vi "ExposeFastConvertNetObjToNumericArray.vi"(11 ".NET Refnum in":refnum<k24>) -> (3 "Array":variant)   [LabVIEW 2017]
uses:
  Mapper/ExposeMapperDataTypeEnum.ctl
  C:/Code/CMCryoSysCode/Expose/COM/CSCom/CSCom/bin/Release/CSCom.dll
  COM/CSCom/CSCom/bin/Release/CSCom.dll
  600bb580-dba4-4572-ab6a-3221339fa0df.vi
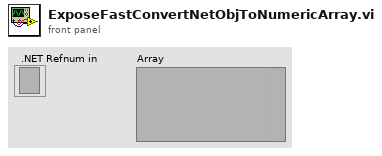
[diagram p1: front panel]
types:
  T1 = typedef "ExposeMapperDataTypeEnum.ctl" = enum16{"NotData", "int8", "byte", "int16", "uint16", "int32", "uint32", "int64", "uint64", "Single", "Double", "String", "Boolean", "Container"}
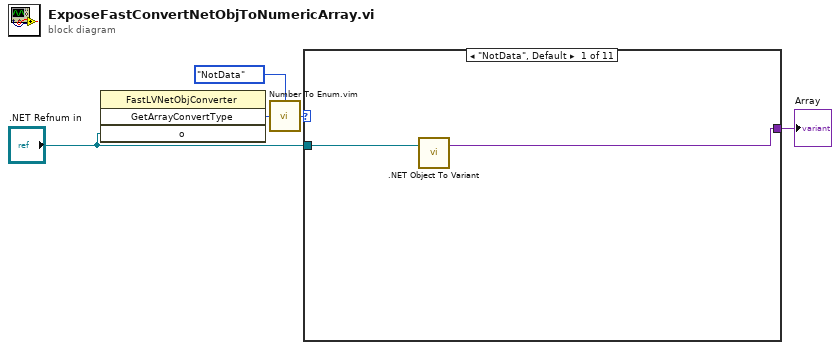
[diagram p0: block diagram]
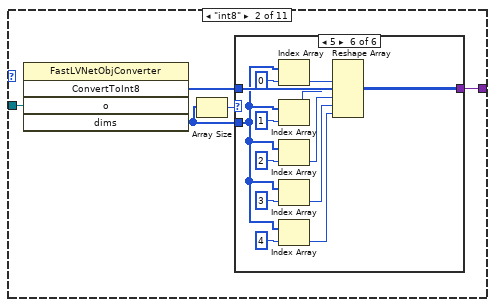
[diagram p2: hidden frame]
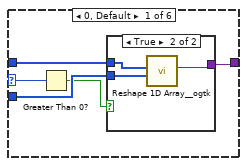
[diagram p3: hidden frame]
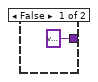
[diagram p4: hidden frame]
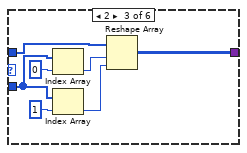
[diagram p6: hidden frame]
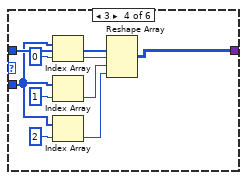
[diagram p7: hidden frame]
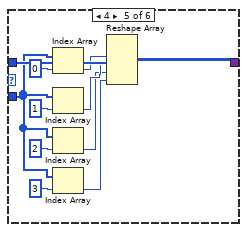
[diagram p8: hidden frame]
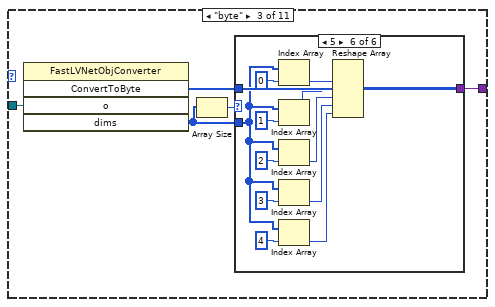
[diagram p9: hidden frame]
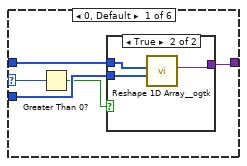
[diagram p10: hidden frame]
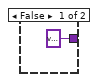
[diagram p11: hidden frame]
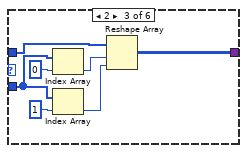
[diagram p13: hidden frame]
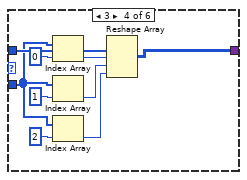
[diagram p14: hidden frame]
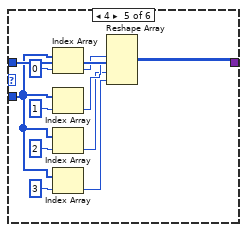
[diagram p15: hidden frame]
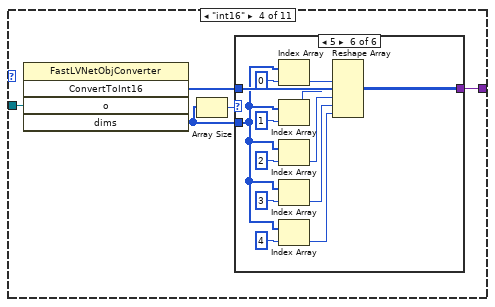
[diagram p16: hidden frame]
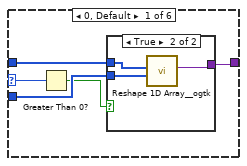
[diagram p17: hidden frame]
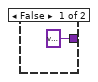
[diagram p18: hidden frame]
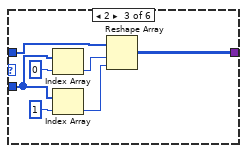
[diagram p20: hidden frame]
diagram:
  n1 = invoke class="FastLVNetObjConverter" method="GetArrayConvertType"("o"=".NET Refnum in") -> ("GetArrayConvertType"=w2:i32)  [unwired: 3 in, 3 out]
  n2 = call "Number To Enum.vim"("number"=w2, "enum type"=ExposeMapperDataTypeEnum."NotData" ("LVPort Matlab Enum")) -> ("number as enum"=w4:T1)
  n3 = case shown="\"NotData\", Default" w4 {
    tunnel: ".NET Refnum in" -> [w7 w12 w67 w122 w177 w232 w287 w342 w397 w452 w507]
    tunnel: [w6 w8 w63 w118 w173 w228 w283 w338 w393 w448 w503] -> w5
    frame "NotData", Default {
      n4 = call <vilib>:".NET Object To Variant.vi"(".NET object"=w7) -> ("variant"=w6:variant)  [unwired: 1 in, 1 out]
    }
    frame "int8" {
      n5 = invoke class="FastLVNetObjConverter" method="ConvertToInt8"("o"=w12) -> ("ConvertToInt8"=w9:i8[], "dims"=w10:i32[])  [unwired: 4 in, 3 out]
      n6 = Array Size(array=w10) -> (size(s)=w11:i32)
      n7 = case shown="5" w11 {
        selector: w11 -> [w17 _ _ _ _ _]
        tunnel: w9 -> [w15 w22 w27 w36 w47 w60]
        tunnel: [w14 w22 w23 w33 w44 w57] -> w8
        tunnel: w10 -> [w16 _ w25 w31 w40 w51]
        frame 0, Default {
          n8 = Greater Than 0?(x=w17) -> (x > 0?=w13:bool)
          n9 = case shown="True" w13 {
            tunnel: w16 -> [_ w21]
            tunnel: w15 -> [_ w20]
            tunnel: [variant w19] -> w14
            frame False {
            }
            frame True {
              n10 = call <userlib>:"Reshape 1D Array__ogtk.vi"("Size(s)"=w21, "1D Array"=w20) -> ("Reshaped VArray"=w19:variant)  [unwired: 8 in, 1 out]
            }
          }
        }
        frame 1 {
        }
        frame 2 {
          n11 = Index Array(array=w25, index=0) -> (element=w24:i32)
          n12 = Index Array(array=w25, index=1) -> (element=w26:i32)
          n13 = Reshape Array(w27, w24, w26) -> (w23:i8[][])
        }
        frame 3 {
          n14 = Index Array(array=w31, index=0) -> (element=w34:i32)
          n15 = Index Array(array=w31, index=1) -> (element=w35:i32)
          n16 = Index Array(array=w31, index=2) -> (element=w30:i32)
          n17 = Reshape Array(w36, w34, w35, w30) -> (w33:i8[][][])
        }
        frame 4 {
          n18 = Index Array(array=w40, index=0) -> (element=w45:i32)
          n19 = Index Array(array=w40, index=1) -> (element=w46:i32)
          n20 = Index Array(array=w40, index=2) -> (element=w42:i32)
          n21 = Index Array(array=w40, index=3) -> (element=w39:i32)
          n22 = Reshape Array(w47, w45, w46, w42, w39) -> (w44:i8[][][][])
        }
        frame 5 {
          n23 = Index Array(array=w51, index=0) -> (element=w58:i32)
          n24 = Index Array(array=w51, index=1) -> (element=w59:i32)
          n25 = Index Array(array=w51, index=2) -> (element=w55:i32)
          n26 = Index Array(array=w51, index=3) -> (element=w53:i32)
          n27 = Index Array(array=w51, index=4) -> (element=w50:i32)
          n28 = Reshape Array(w60, w58, w59, w55, w53, w50) -> (w57:i8[][][][][])
        }
      }
    }
    frame "byte" {
      n29 = invoke class="FastLVNetObjConverter" method="ConvertToByte"("o"=w67) -> ("ConvertToByte"=w64:u8[], "dims"=w65:i32[])  [unwired: 4 in, 3 out]
      n30 = Array Size(array=w65) -> (size(s)=w66:i32)
      n31 = case shown="5" w66 {
        selector: w66 -> [w72 _ _ _ _ _]
        tunnel: w64 -> [w70 w77 w82 w91 w102 w115]
        tunnel: [w69 w77 w78 w88 w99 w112] -> w63
        tunnel: w65 -> [w71 _ w80 w86 w95 w106]
        frame 0, Default {
          n32 = Greater Than 0?(x=w72) -> (x > 0?=w68:bool)
          n33 = case shown="True" w68 {
            tunnel: w71 -> [_ w76]
            tunnel: w70 -> [_ w75]
            tunnel: [variant w74] -> w69
            frame False {
            }
            frame True {
              n34 = call <userlib>:"Reshape 1D Array__ogtk.vi"("Size(s)"=w76, "1D Array"=w75) -> ("Reshaped VArray"=w74:variant)  [unwired: 8 in, 1 out]
            }
          }
        }
        frame 1 {
        }
        frame 2 {
          n35 = Index Array(array=w80, index=0) -> (element=w79:i32)
          n36 = Index Array(array=w80, index=1) -> (element=w81:i32)
          n37 = Reshape Array(w82, w79, w81) -> (w78:u8[][])
        }
        frame 3 {
          n38 = Index Array(array=w86, index=0) -> (element=w89:i32)
          n39 = Index Array(array=w86, index=1) -> (element=w90:i32)
          n40 = Index Array(array=w86, index=2) -> (element=w85:i32)
          n41 = Reshape Array(w91, w89, w90, w85) -> (w88:u8[][][])
        }
        frame 4 {
          n42 = Index Array(array=w95, index=0) -> (element=w100:i32)
          n43 = Index Array(array=w95, index=1) -> (element=w101:i32)
          n44 = Index Array(array=w95, index=2) -> (element=w97:i32)
          n45 = Index Array(array=w95, index=3) -> (element=w94:i32)
          n46 = Reshape Array(w102, w100, w101, w97, w94) -> (w99:u8[][][][])
        }
        frame 5 {
          n47 = Index Array(array=w106, index=0) -> (element=w113:i32)
          n48 = Index Array(array=w106, index=1) -> (element=w114:i32)
          n49 = Index Array(array=w106, index=2) -> (element=w110:i32)
          n50 = Index Array(array=w106, index=3) -> (element=w108:i32)
          n51 = Index Array(array=w106, index=4) -> (element=w105:i32)
          n52 = Reshape Array(w115, w113, w114, w110, w108, w105) -> (w112:u8[][][][][])
        }
      }
    }
    frame "int16" {
      n53 = invoke class="FastLVNetObjConverter" method="ConvertToInt16"("o"=w122) -> ("ConvertToInt16"=w119:i16[], "dims"=w120:i32[])  [unwired: 4 in, 3 out]
      n54 = Array Size(array=w120) -> (size(s)=w121:i32)
      n55 = case shown="5" w121 {
        selector: w121 -> [w127 _ _ _ _ _]
        tunnel: w119 -> [w125 w132 w137 w146 w157 w170]
        tunnel: [w124 w132 w133 w143 w154 w167] -> w118
        tunnel: w120 -> [w126 _ w135 w141 w150 w161]
        frame 0, Default {
          n56 = Greater Than 0?(x=w127) -> (x > 0?=w123:bool)
          n57 = case shown="True" w123 {
            tunnel: w126 -> [_ w131]
            tunnel: w125 -> [_ w130]
            tunnel: [variant w129] -> w124
            frame False {
            }
            frame True {
              n58 = call <userlib>:"Reshape 1D Array__ogtk.vi"("Size(s)"=w131, "1D Array"=w130) -> ("Reshaped VArray"=w129:variant)  [unwired: 8 in, 1 out]
            }
          }
        }
        frame 1 {
        }
        frame 2 {
          n59 = Index Array(array=w135, index=0) -> (element=w134:i32)
          n60 = Index Array(array=w135, index=1) -> (element=w136:i32)
          n61 = Reshape Array(w137, w134, w136) -> (w133:i16[][])
        }
        frame 3 {
          n62 = Index Array(array=w141, index=0) -> (element=w144:i32)
          n63 = Index Array(array=w141, index=1) -> (element=w145:i32)
          n64 = Index Array(array=w141, index=2) -> (element=w140:i32)
          n65 = Reshape Array(w146, w144, w145, w140) -> (w143:i16[][][])
        }
        frame 4 {
          n66 = Index Array(array=w150, index=0) -> (element=w155:i32)
          n67 = Index Array(array=w150, index=1) -> (element=w156:i32)
          n68 = Index Array(array=w150, index=2) -> (element=w152:i32)
          n69 = Index Array(array=w150, index=3) -> (element=w149:i32)
          n70 = Reshape Array(w157, w155, w156, w152, w149) -> (w154:i16[][][][])
        }
        frame 5 {
          n71 = Index Array(array=w161, index=0) -> (element=w168:i32)
          n72 = Index Array(array=w161, index=1) -> (element=w169:i32)
          n73 = Index Array(array=w161, index=2) -> (element=w165:i32)
          n74 = Index Array(array=w161, index=3) -> (element=w163:i32)
          n75 = Index Array(array=w161, index=4) -> (element=w160:i32)
          n76 = Reshape Array(w170, w168, w169, w165, w163, w160) -> (w167:i16[][][][][])
        }
      }
    }
    frame "uint16" {
      n77 = invoke class="FastLVNetObjConverter" method="ConvertToUInt16"("o"=w177) -> ("ConvertToUInt16"=w174:u16[], "dims"=w175:i32[])  [unwired: 4 in, 3 out]
      n78 = Array Size(array=w175) -> (size(s)=w176:i32)
      n79 = case shown="5" w176 {
        selector: w176 -> [w182 _ _ _ _ _]
        tunnel: w174 -> [w180 w187 w192 w201 w212 w225]
        tunnel: [w179 w187 w188 w198 w209 w222] -> w173
        tunnel: w175 -> [w181 _ w190 w196 w205 w216]
        frame 0, Default {
          n80 = Greater Than 0?(x=w182) -> (x > 0?=w178:bool)
          n81 = case shown="True" w178 {
            tunnel: w181 -> [_ w186]
            tunnel: w180 -> [_ w185]
            tunnel: [variant w184] -> w179
            frame False {
            }
            frame True {
              n82 = call <userlib>:"Reshape 1D Array__ogtk.vi"("Size(s)"=w186, "1D Array"=w185) -> ("Reshaped VArray"=w184:variant)  [unwired: 8 in, 1 out]
            }
          }
        }
        frame 1 {
        }
        frame 2 {
          n83 = Index Array(array=w190, index=0) -> (element=w189:i32)
          n84 = Index Array(array=w190, index=1) -> (element=w191:i32)
          n85 = Reshape Array(w192, w189, w191) -> (w188:u16[][])
        }
        frame 3 {
          n86 = Index Array(array=w196, index=0) -> (element=w199:i32)
          n87 = Index Array(array=w196, index=1) -> (element=w200:i32)
          n88 = Index Array(array=w196, index=2) -> (element=w195:i32)
          n89 = Reshape Array(w201, w199, w200, w195) -> (w198:u16[][][])
        }
        frame 4 {
          n90 = Index Array(array=w205, index=0) -> (element=w210:i32)
          n91 = Index Array(array=w205, index=1) -> (element=w211:i32)
          n92 = Index Array(array=w205, index=2) -> (element=w207:i32)
          n93 = Index Array(array=w205, index=3) -> (element=w204:i32)
          n94 = Reshape Array(w212, w210, w211, w207, w204) -> (w209:u16[][][][])
        }
        frame 5 {
          n95 = Index Array(array=w216, index=0) -> (element=w223:i32)
          n96 = Index Array(array=w216, index=1) -> (element=w224:i32)
          n97 = Index Array(array=w216, index=2) -> (element=w220:i32)
          n98 = Index Array(array=w216, index=3) -> (element=w218:i32)
          n99 = Index Array(array=w216, index=4) -> (element=w215:i32)
          n100 = Reshape Array(w225, w223, w224, w220, w218, w215) -> (w222:u16[][][][][])
        }
      }
    }
    frame "int32" {
      n101 = invoke class="FastLVNetObjConverter" method="ConvertToInt32"("o"=w232) -> ("ConvertToInt32"=w229:i32[], "dims"=w230:i32[])  [unwired: 4 in, 3 out]
      n102 = Array Size(array=w230) -> (size(s)=w231:i32)
      n103 = case shown="5" w231 {
        selector: w231 -> [w237 _ _ _ _ _]
        tunnel: w229 -> [w235 w242 w247 w256 w267 w280]
        tunnel: [w234 w242 w243 w253 w264 w277] -> w228
        tunnel: w230 -> [w236 _ w245 w251 w260 w271]
        frame 0, Default {
          n104 = Greater Than 0?(x=w237) -> (x > 0?=w233:bool)
          n105 = case shown="True" w233 {
            tunnel: w236 -> [_ w241]
            tunnel: w235 -> [_ w240]
            tunnel: [variant w239] -> w234
            frame False {
            }
            frame True {
              n106 = call <userlib>:"Reshape 1D Array__ogtk.vi"("Size(s)"=w241, "1D Array"=w240) -> ("Reshaped VArray"=w239:variant)  [unwired: 8 in, 1 out]
            }
          }
        }
        frame 1 {
        }
        frame 2 {
          n107 = Index Array(array=w245, index=0) -> (element=w244:i32)
          n108 = Index Array(array=w245, index=1) -> (element=w246:i32)
          n109 = Reshape Array(w247, w244, w246) -> (w243:i32[][])
        }
        frame 3 {
          n110 = Index Array(array=w251, index=0) -> (element=w254:i32)
          n111 = Index Array(array=w251, index=1) -> (element=w255:i32)
          n112 = Index Array(array=w251, index=2) -> (element=w250:i32)
          n113 = Reshape Array(w256, w254, w255, w250) -> (w253:i32[][][])
        }
        frame 4 {
          n114 = Index Array(array=w260, index=0) -> (element=w265:i32)
          n115 = Index Array(array=w260, index=1) -> (element=w266:i32)
          n116 = Index Array(array=w260, index=2) -> (element=w262:i32)
          n117 = Index Array(array=w260, index=3) -> (element=w259:i32)
          n118 = Reshape Array(w267, w265, w266, w262, w259) -> (w264:i32[][][][])
        }
        frame 5 {
          n119 = Index Array(array=w271, index=0) -> (element=w278:i32)
          n120 = Index Array(array=w271, index=1) -> (element=w279:i32)
          n121 = Index Array(array=w271, index=2) -> (element=w275:i32)
          n122 = Index Array(array=w271, index=3) -> (element=w273:i32)
          n123 = Index Array(array=w271, index=4) -> (element=w270:i32)
          n124 = Reshape Array(w280, w278, w279, w275, w273, w270) -> (w277:i32[][][][][])
        }
      }
    }
    frame "uint32" {
      n125 = invoke class="FastLVNetObjConverter" method="ConvertToUInt32"("o"=w287) -> ("ConvertToUInt32"=w284:u32[], "dims"=w285:i32[])  [unwired: 4 in, 3 out]
      n126 = Array Size(array=w285) -> (size(s)=w286:i32)
      n127 = case shown="5" w286 {
        selector: w286 -> [w292 _ _ _ _ _]
        tunnel: w284 -> [w290 w297 w302 w311 w322 w335]
        tunnel: [w289 w297 w298 w308 w319 w332] -> w283
        tunnel: w285 -> [w291 _ w300 w306 w315 w326]
        frame 0, Default {
          n128 = Greater Than 0?(x=w292) -> (x > 0?=w288:bool)
          n129 = case shown="True" w288 {
            tunnel: w291 -> [_ w296]
            tunnel: w290 -> [_ w295]
            tunnel: [variant w294] -> w289
            frame False {
            }
            frame True {
              n130 = call <userlib>:"Reshape 1D Array__ogtk.vi"("Size(s)"=w296, "1D Array"=w295) -> ("Reshaped VArray"=w294:variant)  [unwired: 8 in, 1 out]
            }
          }
        }
        frame 1 {
        }
        frame 2 {
          n131 = Index Array(array=w300, index=0) -> (element=w299:i32)
          n132 = Index Array(array=w300, index=1) -> (element=w301:i32)
          n133 = Reshape Array(w302, w299, w301) -> (w298:u32[][])
        }
        frame 3 {
          n134 = Index Array(array=w306, index=0) -> (element=w309:i32)
          n135 = Index Array(array=w306, index=1) -> (element=w310:i32)
          n136 = Index Array(array=w306, index=2) -> (element=w305:i32)
          n137 = Reshape Array(w311, w309, w310, w305) -> (w308:u32[][][])
        }
        frame 4 {
          n138 = Index Array(array=w315, index=0) -> (element=w320:i32)
          n139 = Index Array(array=w315, index=1) -> (element=w321:i32)
          n140 = Index Array(array=w315, index=2) -> (element=w317:i32)
          n141 = Index Array(array=w315, index=3) -> (element=w314:i32)
          n142 = Reshape Array(w322, w320, w321, w317, w314) -> (w319:u32[][][][])
        }
        frame 5 {
          n143 = Index Array(array=w326, index=0) -> (element=w333:i32)
          n144 = Index Array(array=w326, index=1) -> (element=w334:i32)
          n145 = Index Array(array=w326, index=2) -> (element=w330:i32)
          n146 = Index Array(array=w326, index=3) -> (element=w328:i32)
          n147 = Index Array(array=w326, index=4) -> (element=w325:i32)
          n148 = Reshape Array(w335, w333, w334, w330, w328, w325) -> (w332:u32[][][][][])
        }
      }
    }
    frame "int64" {
      n149 = invoke class="FastLVNetObjConverter" method="ConvertToInt64"("o"=w342) -> ("ConvertToInt64"=w339:i64[], "dims"=w340:i32[])  [unwired: 4 in, 3 out]
      n150 = Array Size(array=w340) -> (size(s)=w341:i32)
      n151 = case shown="5" w341 {
        selector: w341 -> [w347 _ _ _ _ _]
        tunnel: w339 -> [w345 w352 w357 w366 w377 w390]
        tunnel: [w344 w352 w353 w363 w374 w387] -> w338
        tunnel: w340 -> [w346 _ w355 w361 w370 w381]
        frame 0, Default {
          n152 = Greater Than 0?(x=w347) -> (x > 0?=w343:bool)
          n153 = case shown="True" w343 {
            tunnel: w346 -> [_ w351]
            tunnel: w345 -> [_ w350]
            tunnel: [variant w349] -> w344
            frame False {
            }
            frame True {
              n154 = call <userlib>:"Reshape 1D Array__ogtk.vi"("Size(s)"=w351, "1D Array"=w350) -> ("Reshaped VArray"=w349:variant)  [unwired: 8 in, 1 out]
            }
          }
        }
        frame 1 {
        }
        frame 2 {
          n155 = Index Array(array=w355, index=0) -> (element=w354:i32)
          n156 = Index Array(array=w355, index=1) -> (element=w356:i32)
          n157 = Reshape Array(w357, w354, w356) -> (w353:i64[][])
        }
        frame 3 {
          n158 = Index Array(array=w361, index=0) -> (element=w364:i32)
          n159 = Index Array(array=w361, index=1) -> (element=w365:i32)
          n160 = Index Array(array=w361, index=2) -> (element=w360:i32)
          n161 = Reshape Array(w366, w364, w365, w360) -> (w363:i64[][][])
        }
        frame 4 {
          n162 = Index Array(array=w370, index=0) -> (element=w375:i32)
          n163 = Index Array(array=w370, index=1) -> (element=w376:i32)
          n164 = Index Array(array=w370, index=2) -> (element=w372:i32)
          n165 = Index Array(array=w370, index=3) -> (element=w369:i32)
          n166 = Reshape Array(w377, w375, w376, w372, w369) -> (w374:i64[][][][])
        }
        frame 5 {
          n167 = Index Array(array=w381, index=0) -> (element=w388:i32)
          n168 = Index Array(array=w381, index=1) -> (element=w389:i32)
          n169 = Index Array(array=w381, index=2) -> (element=w385:i32)
          n170 = Index Array(array=w381, index=3) -> (element=w383:i32)
          n171 = Index Array(array=w381, index=4) -> (element=w380:i32)
          n172 = Reshape Array(w390, w388, w389, w385, w383, w380) -> (w387:i64[][][][][])
        }
      }
    }
    frame "uint64" {
      n173 = invoke class="FastLVNetObjConverter" method="ConvertToUInt64"("o"=w397) -> ("ConvertToUInt64"=w394:u64[], "dims"=w395:i32[])  [unwired: 4 in, 3 out]
      n174 = Array Size(array=w395) -> (size(s)=w396:i32)
      n175 = case shown="5" w396 {
        selector: w396 -> [w402 _ _ _ _ _]
        tunnel: w394 -> [w400 w407 w412 w421 w432 w445]
        tunnel: [w399 w407 w408 w418 w429 w442] -> w393
        tunnel: w395 -> [w401 _ w410 w416 w425 w436]
        frame 0, Default {
          n176 = Greater Than 0?(x=w402) -> (x > 0?=w398:bool)
          n177 = case shown="True" w398 {
            tunnel: w401 -> [_ w406]
            tunnel: w400 -> [_ w405]
            tunnel: [variant w404] -> w399
            frame False {
            }
            frame True {
              n178 = call <userlib>:"Reshape 1D Array__ogtk.vi"("Size(s)"=w406, "1D Array"=w405) -> ("Reshaped VArray"=w404:variant)  [unwired: 8 in, 1 out]
            }
          }
        }
        frame 1 {
        }
        frame 2 {
          n179 = Index Array(array=w410, index=0) -> (element=w409:i32)
          n180 = Index Array(array=w410, index=1) -> (element=w411:i32)
          n181 = Reshape Array(w412, w409, w411) -> (w408:u64[][])
        }
        frame 3 {
          n182 = Index Array(array=w416, index=0) -> (element=w419:i32)
          n183 = Index Array(array=w416, index=1) -> (element=w420:i32)
          n184 = Index Array(array=w416, index=2) -> (element=w415:i32)
          n185 = Reshape Array(w421, w419, w420, w415) -> (w418:u64[][][])
        }
        frame 4 {
          n186 = Index Array(array=w425, index=0) -> (element=w430:i32)
          n187 = Index Array(array=w425, index=1) -> (element=w431:i32)
          n188 = Index Array(array=w425, index=2) -> (element=w427:i32)
          n189 = Index Array(array=w425, index=3) -> (element=w424:i32)
          n190 = Reshape Array(w432, w430, w431, w427, w424) -> (w429:u64[][][][])
        }
        frame 5 {
          n191 = Index Array(array=w436, index=0) -> (element=w443:i32)
          n192 = Index Array(array=w436, index=1) -> (element=w444:i32)
          n193 = Index Array(array=w436, index=2) -> (element=w440:i32)
          n194 = Index Array(array=w436, index=3) -> (element=w438:i32)
          n195 = Index Array(array=w436, index=4) -> (element=w435:i32)
          n196 = Reshape Array(w445, w443, w444, w440, w438, w435) -> (w442:u64[][][][][])
        }
      }
    }
    frame "Single" {
      n197 = invoke class="FastLVNetObjConverter" method="ConvertToSingle"("o"=w452) -> ("ConvertToSingle"=w449:sgl[], "dims"=w450:i32[])  [unwired: 4 in, 3 out]
      n198 = Array Size(array=w450) -> (size(s)=w451:i32)
      n199 = case shown="5" w451 {
        selector: w451 -> [w457 _ _ _ _ _]
        tunnel: w449 -> [w455 w462 w467 w476 w487 w500]
        tunnel: [w454 w462 w463 w473 w484 w497] -> w448
        tunnel: w450 -> [w456 _ w465 w471 w480 w491]
        frame 0, Default {
          n200 = Greater Than 0?(x=w457) -> (x > 0?=w453:bool)
          n201 = case shown="True" w453 {
            tunnel: w456 -> [_ w461]
            tunnel: w455 -> [_ w460]
            tunnel: [variant w459] -> w454
            frame False {
            }
            frame True {
              n202 = call <userlib>:"Reshape 1D Array__ogtk.vi"("Size(s)"=w461, "1D Array"=w460) -> ("Reshaped VArray"=w459:variant)  [unwired: 8 in, 1 out]
            }
          }
        }
        frame 1 {
        }
        frame 2 {
          n203 = Index Array(array=w465, index=0) -> (element=w464:i32)
          n204 = Index Array(array=w465, index=1) -> (element=w466:i32)
          n205 = Reshape Array(w467, w464, w466) -> (w463:sgl[][])
        }
        frame 3 {
          n206 = Index Array(array=w471, index=0) -> (element=w474:i32)
          n207 = Index Array(array=w471, index=1) -> (element=w475:i32)
          n208 = Index Array(array=w471, index=2) -> (element=w470:i32)
          n209 = Reshape Array(w476, w474, w475, w470) -> (w473:sgl[][][])
        }
        frame 4 {
          n210 = Index Array(array=w480, index=0) -> (element=w485:i32)
          n211 = Index Array(array=w480, index=1) -> (element=w486:i32)
          n212 = Index Array(array=w480, index=2) -> (element=w482:i32)
          n213 = Index Array(array=w480, index=3) -> (element=w479:i32)
          n214 = Reshape Array(w487, w485, w486, w482, w479) -> (w484:sgl[][][][])
        }
        frame 5 {
          n215 = Index Array(array=w491, index=0) -> (element=w498:i32)
          n216 = Index Array(array=w491, index=1) -> (element=w499:i32)
          n217 = Index Array(array=w491, index=2) -> (element=w495:i32)
          n218 = Index Array(array=w491, index=3) -> (element=w493:i32)
          n219 = Index Array(array=w491, index=4) -> (element=w490:i32)
          n220 = Reshape Array(w500, w498, w499, w495, w493, w490) -> (w497:sgl[][][][][])
        }
      }
    }
    frame "Double" {
      n221 = invoke class="FastLVNetObjConverter" method="ConvertToDouble"("o"=w507) -> ("ConvertToDouble"=w504:dbl[], "dims"=w505:i32[])  [unwired: 4 in, 3 out]
      n222 = Array Size(array=w505) -> (size(s)=w506:i32)
      n223 = case shown="5" w506 {
        selector: w506 -> [w512 _ _ _ _ _]
        tunnel: w504 -> [w510 w517 w522 w531 w542 w555]
        tunnel: [w509 w517 w518 w528 w539 w552] -> w503
        tunnel: w505 -> [w511 _ w520 w526 w535 w546]
        frame 0, Default {
          n224 = Greater Than 0?(x=w512) -> (x > 0?=w508:bool)
          n225 = case shown="True" w508 {
            tunnel: w511 -> [_ w516]
            tunnel: w510 -> [_ w515]
            tunnel: [variant w514] -> w509
            frame False {
            }
            frame True {
              n226 = call <userlib>:"Reshape 1D Array__ogtk.vi"("Size(s)"=w516, "1D Array"=w515) -> ("Reshaped VArray"=w514:variant)  [unwired: 8 in, 1 out]
            }
          }
        }
        frame 1 {
        }
        frame 2 {
          n227 = Index Array(array=w520, index=0) -> (element=w519:i32)
          n228 = Index Array(array=w520, index=1) -> (element=w521:i32)
          n229 = Reshape Array(w522, w519, w521) -> (w518:dbl[][])
        }
        frame 3 {
          n230 = Index Array(array=w526, index=0) -> (element=w529:i32)
          n231 = Index Array(array=w526, index=1) -> (element=w530:i32)
          n232 = Index Array(array=w526, index=2) -> (element=w525:i32)
          n233 = Reshape Array(w531, w529, w530, w525) -> (w528:dbl[][][])
        }
        frame 4 {
          n234 = Index Array(array=w535, index=0) -> (element=w540:i32)
          n235 = Index Array(array=w535, index=1) -> (element=w541:i32)
          n236 = Index Array(array=w535, index=2) -> (element=w537:i32)
          n237 = Index Array(array=w535, index=3) -> (element=w534:i32)
          n238 = Reshape Array(w542, w540, w541, w537, w534) -> (w539:dbl[][][][])
        }
        frame 5 {
          n239 = Index Array(array=w546, index=0) -> (element=w553:i32)
          n240 = Index Array(array=w546, index=1) -> (element=w554:i32)
          n241 = Index Array(array=w546, index=2) -> (element=w550:i32)
          n242 = Index Array(array=w546, index=3) -> (element=w548:i32)
          n243 = Index Array(array=w546, index=4) -> (element=w545:i32)
          n244 = Reshape Array(w555, w553, w554, w550, w548, w545) -> (w552:dbl[][][][][])
        }
      }
    }
  }
  "Array" <- w5
